vi "newPassword.vi"(11 "Username":string) -> ()   [LabVIEW 2020, in "userLibrary.lvlib"]
uses:
  userLibrary.lvlib
  <vilib>/measure/mamon.llb/Trigger Detection for 1 Channel.vi
  <vilib>/addons/database/Connection.llb/DB Tools Open Connec (String).vi
  <vilib>/addons/database/_DB Variant To Data/Database Variant To Data.xnode
  <vilib>/addons/database/NI_Database_API.lvlib
  maintenanceLibrary.lvlib
  <vilib>/measure/NI_MAPro.lvlib
  databaseLibrary.lvlib
panel:
  out "status 2":bool
  out "status 1":bool
  out "Log Max row":i32
  in  "Cancel":bool
  in  "OK":bool
  in  "Old Password":string
  in  "Confirm New Password":string
  in  "New Password":string
  out "Username 2":string caption="Username"
  # "New Password"
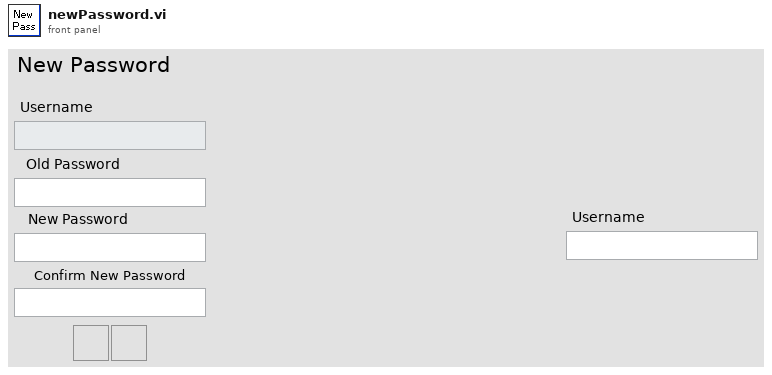
[diagram p1: front panel]
types:
  T1 = typedef "NI_Database_API.lvlib/Conn ObjectReference.ctl" = refnum<k1>
  T2 = cluster{"table":string, "date/time string":string, "date/time string":string, string}
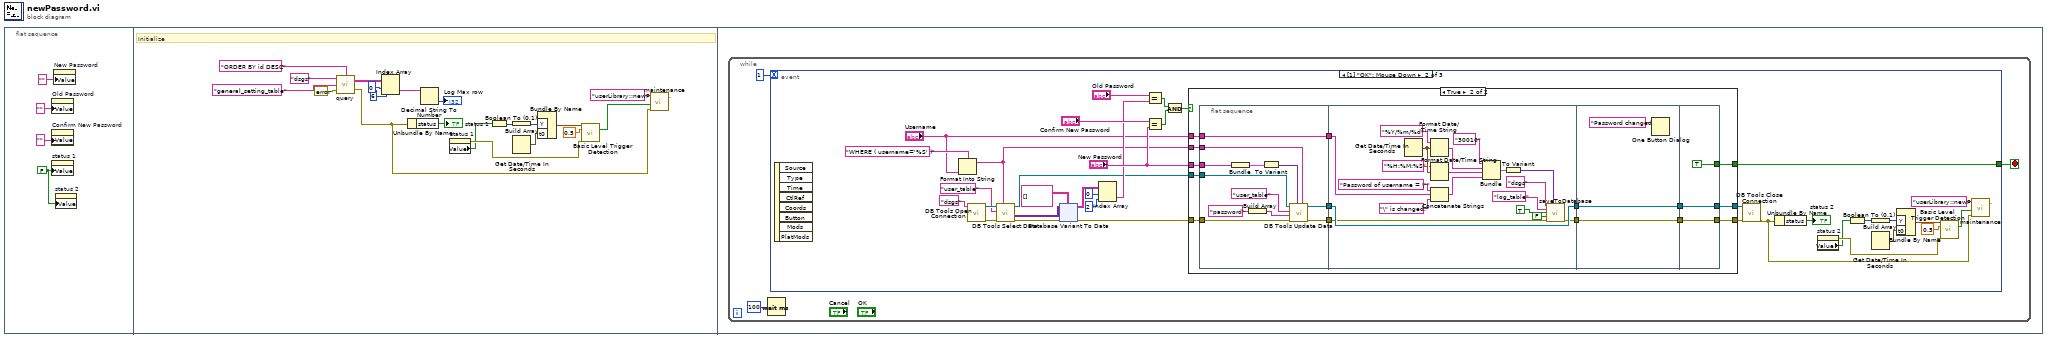
[diagram p0: block diagram]
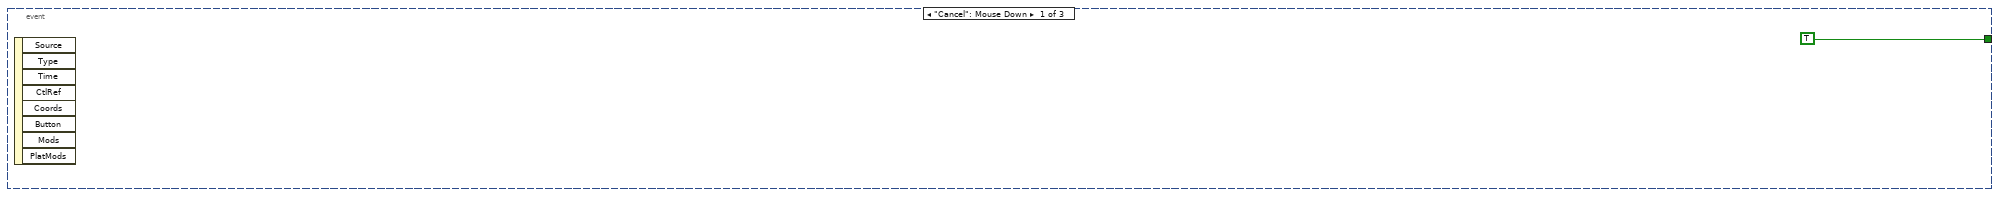
[diagram p2: hidden frame]
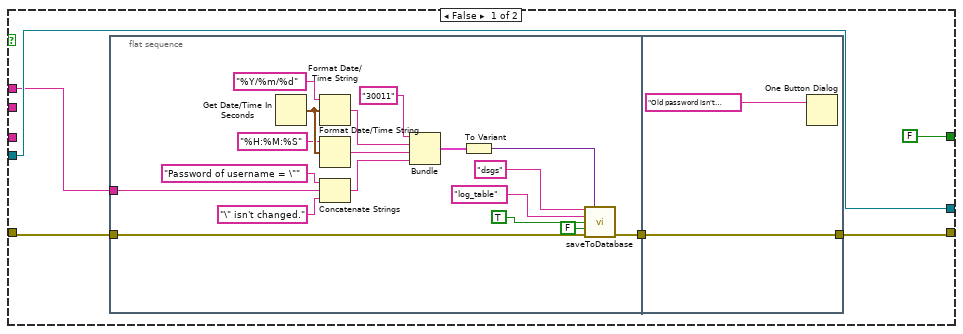
[diagram p3: hidden frame]
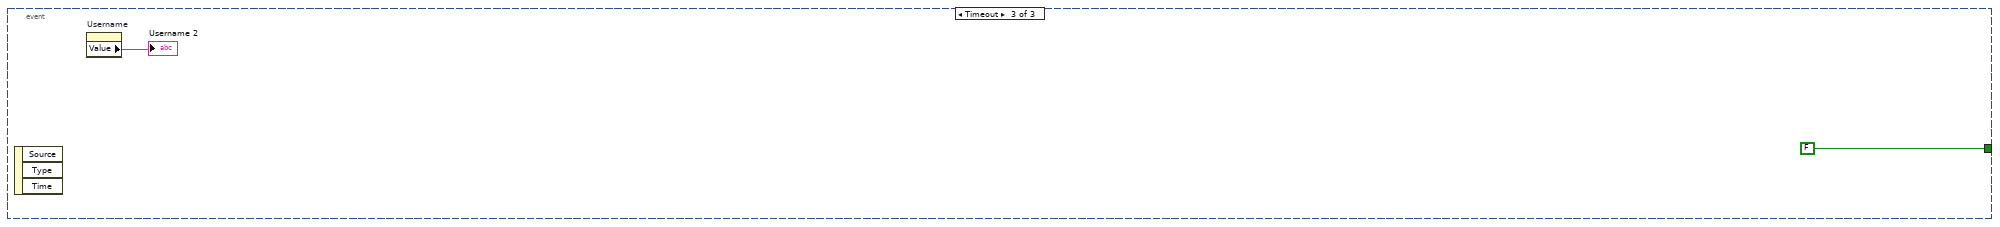
[diagram p4: hidden frame]
diagram:
  n1 = flat-sequence {
    frame #0 {
      w1 = FALSE ("status 1")
      n2 = property on="Old Password" class="Str"("Value"="" ("New Password")) -> ()  [unwired: 2 in, 2 out]
      n3 = property on="Confirm New Password" class="Str"("Value"="" ("New Password")) -> ()  [unwired: 2 in, 2 out]
      n4 = property on="status 1" class="Bool (strict)"("Value"=w1) -> ()  [unwired: 2 in, 2 out]
      n5 = property on="New Password" class="Str"("Value"="" ("New Password")) -> ()  [unwired: 2 in, 2 out]
      n6 = property on="status 2" class="Bool (strict)"("Value"=w1) -> ()  [unwired: 2 in, 2 out]
    }
    frame #1 {
      # "Initialize"
      n7 = call "query.vi"("Condition"="ORDER BY id DESC", "errorIn"=errorcluster {"status"=FALSE, "code"=0, "source"=""} ("Error in"), "Table Name"="general_setting_table", "Connection Name"="dsgs") -> ("errorOut"=w7:errorcluster, "data"=w24:string[][])
      n8 = Index Array(array=w24, index (row)=0, index (col)=6 ("disabled index (col)")) -> (element=w5:string)
      n9 = Unbundle By Name(w7) -> ("status"=→"status 1":bool)
      n10 = Decimal String To Number(string=w5) -> (number=→"Log Max row":i32)  [unwired: 2 in, 1 out]
      n11 = property on="status 1" class="Bool (strict)"() -> (error out=w15:errorcluster, "Value"=w14:bool)  [unwired: 2 in, 1 out]
      n12 = Boolean To (0,1)(Boolean=w14) -> (0, 1=w10:i16)
      n13 = Build Array(w10) -> (w12:i16[])
      n14 = Get Date/Time In Seconds() -> (seconds since 1Jan1904=w11:timestamp)
      n15 = Bundle By Name("Y"=w12, "t0"=w11) -> (w13:waveform(i16))  [unwired: 1 in]
      n16 = call-poly <vilib>:"Basic Level Trigger Detection.vi"("signal in"=w13, "level"=0.5, "error in (no error)"=w15) -> ("trigger detected?"=w16:bool)  [unwired: 10 in, 2 out]
      n17 = call "maintenance.vi"("errorIn"=w7, "status"=w16, "errorLocation"="userLibrary::newPassword.vi::Initialize") -> ()  [unwired: 8 in, 1 out]
    }
    frame #2 {
      n18 = while {
        stop <- w26 stop-if-true
        n19 = Wait (ms)(milliseconds to wait=u32 100) -> ()  [unwired: 1 out]
        n20 = event shown="[1] \"OK\": Mouse Down" {
          selector: _ -> [_ _ _]
          dyn-events: _ -> [_ _ _]
          timeout: 1 -> [_ _ _]
          tunnel: [TRUE w40 FALSE] -> w26
          event "Cancel": Mouse Down {
            n21 = event-data() -> ()  [unwired: 1 in, 8 out]
          }
          event "OK": Mouse Down {
            n22 = event-data() -> ()  [unwired: 1 in, 8 out]
            n23 = Format Into String(format string="WHERE ( username='%S' )" ("condition"), "Username") -> (resulting string=w53:string)  [unwired: 2 in, 1 out]
            n24 = call-poly <vilib>:"DB Tools Open Connection.vi"("connection information"="dsgs") -> ("error out"=w48:errorcluster, "connection reference"=w49:T1)  [unwired: 7 in]
            n25 = call <vilib>:"DB Tools Select Data.vi"("condition"=w53, "error in (no error)"=w48, "table"="user_table", "connection reference"=w49) -> ("error out"=w55:errorcluster, "data"=w54:variant[][], "connection reference out"=w50:T1)  [unwired: 2 in]
            n26 = xnode "Database Variant To Data"("database variant"=w54, "error in (no error)"=w55, "type"=string[][] []) -> ("data"=w57:string[][], "error out"=w56:errorcluster)
            n27 = Index Array(array=w57, index (row)=0 ("disabled index (row)"), index (col)=2 ("disabled index (col)")) -> (element=w58:string)
            n28 = Equal?(x="Old Password", y=w58) -> (x = y?=w59:bool)
            n29 = Equal?(x="Confirm New Password", y="New Password") -> (x = y?=w60:bool)
            n30 = And(x=w59, y=w60) -> (x .and. y?=w61:bool)
            n31 = case shown="True" w61 {
              tunnel: w53 -> [_ w149]
              tunnel: "New Password" -> [_ w148]
              tunnel: w56 -> [w112 w146]
              tunnel: w50 -> [w114 w147]
              tunnel: [w111 w145] -> w51
              tunnel: [w114 w144] -> w52
              tunnel: [FALSE w137] -> w40
              tunnel: "Username" -> [w110 w135]
              frame False {
                n32 = flat-sequence {
                  tunnel: w112 -> [w118]
                  tunnel: w110 -> [w116]
                  tunnel: [w117] -> w109
                  tunnel: [w134] -> w111
                  tunnel: w109 -> [w134]
                  frame #0 {
                    n33 = Get Date/Time In Seconds() -> (seconds since 1Jan1904=w128:timestamp)
                    n34 = Format Date/Time String(time format string (%c)="%Y/%m/%d", seconds (now)=w128) -> (date/time string=w129:string)  [unwired: 1 in]
                    n35 = Format Date/Time String(time format string (%c)="%H:%M:%S", seconds (now)=w128) -> (date/time string=w130:string)  [unwired: 1 in]
                    n36 = Concatenate Strings("Password of username = \"" ("string"), w116, "\" isn't changed." ("string")) -> (w122:string)
                    n37 = Bundle("table"="30011", "date/time string"=w129, "date/time string"=w130, w122) -> (w131:T2)  [unwired: 1 in]
                    n38 = To Variant(anything=w131) -> (Variant=w132:variant)
                    n39 = call "saveToDatabase.vi"("Connection"="dsgs" ("table"), "Data"=w132, "Table"="log_table" ("table"), "Auto Increment ID?"=TRUE, "Delete row?"=FALSE, "Error in"=w118) -> ("Error out"=w117:errorcluster)  [unwired: 9 in]
                  }
                  frame #1 {
                    n40 = One Button Dialog(message="Old password isn't correct or new password does not confirm.") -> ()  [unwired: 1 in, 1 out]
                  }
                }
              }
              frame True {
                n41 = flat-sequence {
                  tunnel: w149 -> [w159]
                  tunnel: w148 -> [w157]
                  tunnel: w147 -> [w154]
                  tunnel: w146 -> [w153]
                  tunnel: [w152] -> w143
                  tunnel: [w151] -> w142
                  tunnel: [w150] -> w136
                  tunnel: w135 -> [w150]
                  tunnel: w143 -> [w170]
                  tunnel: w142 -> [w180]
                  tunnel: [w169] -> w141
                  tunnel: [w180] -> w140
                  tunnel: w136 -> [w167]
                  tunnel: w141 -> [w183]
                  tunnel: w140 -> [w182]
                  tunnel: [w183] -> w139
                  tunnel: [w182] -> w138
                  tunnel: [w185] -> w144
                  tunnel: [w186] -> w145
                  tunnel: w139 -> [w186]
                  tunnel: w138 -> [w185]
                  tunnel: [TRUE] -> w137
                  frame #0 {
                    n42 = Bundle("New Password"=w157) -> (w156:cluster{"New Password":string})  [unwired: 1 in]
                    n43 = Build Array("password" ("table")) -> (w161:string[])
                    n44 = To Variant(anything=w156) -> (Variant=w155:variant)
                    n45 = call <vilib>:"DB Tools Update Data.vi"("condition"=w159, "data"=w155, "error in (no error)"=w153, "columns"=w161, "table"="user_table", "connection reference"=w154) -> ("error out"=w152:errorcluster, "connection reference out"=w151:T1)  [unwired: 4 in]
                  }
                  frame #1 {
                    n46 = Get Date/Time In Seconds() -> (seconds since 1Jan1904=w175:timestamp)
                    n47 = Format Date/Time String(time format string (%c)="%Y/%m/%d", seconds (now)=w175) -> (date/time string=w176:string)  [unwired: 1 in]
                    n48 = Format Date/Time String(time format string (%c)="%H:%M:%S", seconds (now)=w175) -> (date/time string=w177:string)  [unwired: 1 in]
                    n49 = Concatenate Strings("Password of username = \"" ("string"), w167, "\" is changed." ("string")) -> (w166:string)
                    n50 = Bundle("table"="30010", "date/time string"=w176, "date/time string"=w177, w166) -> (w178:T2)  [unwired: 1 in]
                    n51 = To Variant(anything=w178) -> (Variant=w179:variant)
                    n52 = call "saveToDatabase.vi"("Connection"="dsgs" ("table"), "Data"=w179, "Table"="log_table" ("table"), "Auto Increment ID?"=TRUE, "Delete row?"=FALSE, "Error in"=w170) -> ("Error out"=w169:errorcluster)  [unwired: 9 in]
                  }
                  frame #2 {
                    n53 = One Button Dialog(message="Password changed.") -> ()  [unwired: 1 in, 1 out]
                  }
                  frame #3 {
                  }
                }
              }
            }
            n54 = call <vilib>:"DB Tools Close Connection.vi"("error in (no error)"=w51, "connection reference"=w52) -> ("error out"=w29:errorcluster)  [unwired: 5 in]
            n55 = Unbundle By Name(w29) -> ("status"=→"status 2":bool)
            n56 = property on="status 2" class="Bool (strict)"() -> (error out=w37:errorcluster, "Value"=w36:bool)  [unwired: 2 in, 1 out]
            n57 = Boolean To (0,1)(Boolean=w36) -> (0, 1=w32:i16)
            n58 = Build Array(w32) -> (w34:i16[])
            n59 = Get Date/Time In Seconds() -> (seconds since 1Jan1904=w33:timestamp)
            n60 = Bundle By Name("Y"=w34, "t0"=w33) -> (w35:waveform(i16))  [unwired: 1 in]
            n61 = call-poly <vilib>:"Basic Level Trigger Detection.vi"("signal in"=w35, "level"=0.5, "error in (no error)"=w37) -> ("trigger detected?"=w38:bool)  [unwired: 10 in, 2 out]
            n62 = call "maintenance.vi"("errorIn"=w29, "status"=w38, "errorLocation"="userLibrary::newPassword.vi::OK case") -> ()  [unwired: 8 in, 1 out]
          }
          event Timeout {
            n63 = event-data() -> ()  [unwired: 1 in, 3 out]
            n64 = property on="Username" class="Str"() -> ("Value"=→"Username 2":string)  [unwired: 2 in, 2 out]
          }
        }
      }
    }
  }
